vi "start.vi"() -> (3 "function return":i32)   [LabVIEW 2017, in "HapticSTM.lvlib"]
doc: "extern \"C\" __declspec(dllexport) int start();"
uses:
  <userlib>/HapticSTM/Feedbackless - Testdata/Project/feedbackless.lvproj/Proj/Feedbackless Folder/HapticSTM/HapticSTM.lvlib
  <userlib>/HapticSTM/HapticSTM.dll
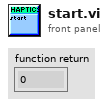
[diagram p1: front panel]
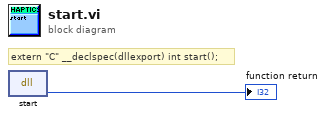
[diagram p0: block diagram]
diagram:
  # "extern \"C\" __declspec(dllexport) int start();"
  n1 = dll-call lib="C:/Program Files/National Instruments/LabVIEW 2017/user.lib/HapticSTM/HapticSTM.*" fn="start"() -> (→"function return":i32)  [unwired: 3 in, 2 out]
